vi "2 wind_degree_shift.vi"(1 "Wind Vector -180 - 180":cluster{"Wind Speed":dbl, "Wind Theta":dbl}) -> (0 "Wind Vector 0-360":cluster{"Wind Speed":dbl, "Wind Theta":dbl})   [LabVIEW 2011]
doc: "Changes wind range from [-180:180] to [0:360]"
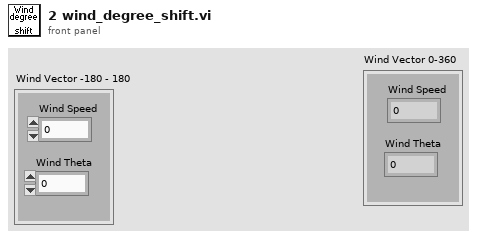
[diagram p1: front panel]
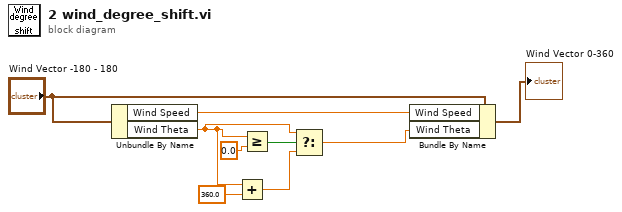
[diagram p0: block diagram]
diagram:
  n1 = Unbundle By Name("Wind Vector -180 - 180") -> ("Wind Speed"=w8:dbl, "Wind Theta"=w4:dbl)
  n2 = Add(x=w4, y=360.0) -> (x+y=w2:dbl)
  n3 = Greater Or Equal?(x=w4, y=0.0) -> (x >= y?=w6:bool)
  n4 = Select(t=w4, s=w6, f=w2) -> (s? t:f=w5:dbl)
  n5 = Bundle By Name(cluster="Wind Vector -180 - 180", "Wind Speed"=w8, "Wind Theta"=w5) -> (→"Wind Vector 0-360":cluster{"Wind Speed":dbl, "Wind Theta":dbl})
